vi "StartAsyncWorker.vi"(8 "error in (no error)":errorcluster, 10 "ResultProcessor Config.lvclass":refnum<class "ResultProcessor Config.lvclass">, 11 "ResultProcessor in":refnum<class "ResultProcessor.lvclass">) -> (0 "error out":errorcluster, 3 "ResultProcessor out":refnum<class "ResultProcessor.lvclass">)   [LabVIEW 2015, in "ResultProcessor.lvclass"]
doc: "This VI creates the communication queue and starts the result processor asynchronously."
uses:
  ResultProcessor.lvclass
  Config/ResultProcessor Config.lvclass
  CommandQueueDataType.ctl
  Report Information/Report Information.lvclass
  Result/Result.lvclass
  ErrorQueueDataType.ctl
  ResultProcessor.lvclass/ResultProcessor.ctl
  AsyncWorker.vi
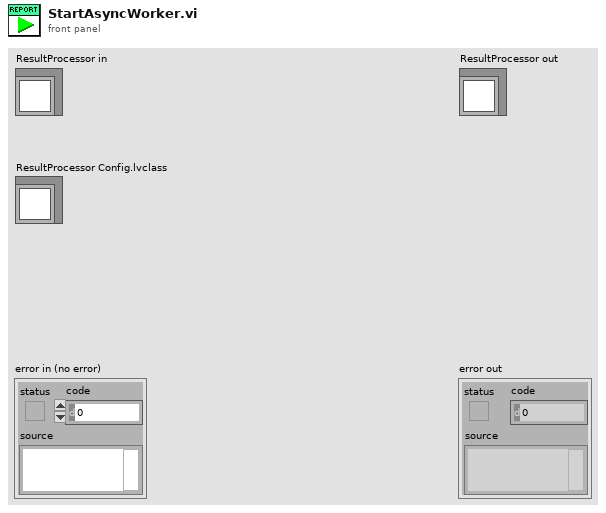
[diagram p1: front panel]
types:
  T1 = typedef "ResultProcessor.lvclass/ErrorQueueDataType.ctl" = cluster{"error out":errorcluster}
  T2 = typedef "ResultProcessor.lvclass/CommandQueueDataType.ctl" = cluster{"Command":enum16{"New Report", "Add Result", "Publish Report", "Shutdown", "Add DUT Information", "Add Station Information", "Add Report Information", "Add Test Information"}, "Report Information.lvclass":refnum<class "Report Information.lvclass">, "Result.lvclass":refnum<class "Result.lvclass">}
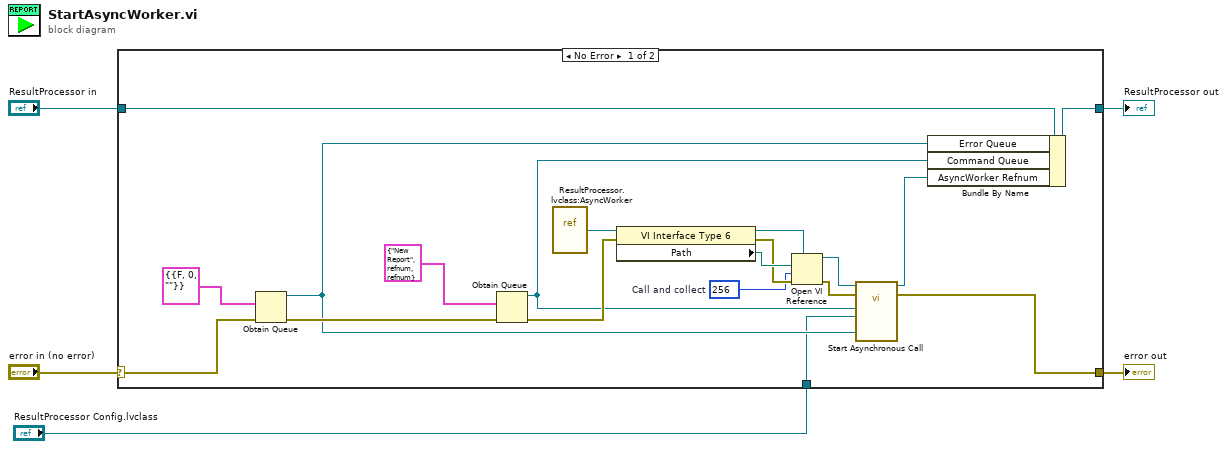
[diagram p0: block diagram]
diagram:
  n1 = case shown="No Error" "error in (no error)" {
    selector: "error in (no error)" -> [w8 w26]
    tunnel: [w12 w26] -> w4
    tunnel: [w22 w25] -> w2
    tunnel: "ResultProcessor in" -> [w24 w25]
    tunnel: "ResultProcessor Config.lvclass" -> [w6 _]
    frame No Error {
      w14 = 256  # Call and collect
      n2 = Obtain Queue(element data type=T1 {"error out"={"status"=FALSE, "code"=0, "source"=""}} ("Cluster"), error in (no error)=w8) -> (queue out=w7:refnum<queue>, error out=w9:errorcluster)  [unwired: 3 in, 1 out]
      n3 = Obtain Queue(element data type=T2 {"Command"=enum."New Report", "Report Information.lvclass"=refnum, "Result.lvclass"=refnum}, error in (no error)=w9) -> (queue out=w13:refnum<queue>, error out=w15:errorcluster)  [unwired: 3 in, 1 out]
      n4 = vi-ref "ResultProcessor.lvclass:AsyncWorker.vi"() -> (w18:refnum<vi>)
      n5 = property class="VI Interface Type 6"(reference=w18, error in=w15) -> (reference out=w21:refnum<vi>, error out=w16:errorcluster, "Path"=w20:path)
      n6 = Open VI Reference(type specifier VI Refnum (for type only)=w21, vi path=w20, options=w14, error in (no error)=w16) -> (vi reference=w19:refnum<vi>, error out=w17:errorcluster)  [unwired: 2 in]
      n7 = call-by-ref "Start Asynchronous Call"(reference=w19, error in=w17, "Error Queue"=w7, "ResultProcessor Config.lvclass"=w6, "Command Queue"=w13) -> (reference out=w11:refnum<vi>, error out=w12:errorcluster)  [unwired: 9 in]
      n8 = Bundle By Name(cluster=w24, "Error Queue"=w7, "Command Queue"=w13, "AsyncWorker Refnum"=w11) -> (w22:refnum<class "ResultProcessor.lvclass">)
    }
    frame Error {
    }
  }
  "error out" <- w4
  "ResultProcessor out" <- w2
